vi "Sample Trajectory.vi"(9 "start index (0)":i32, 10 "timestamp":dbl, 11 "Trajectory States":T1[](array[typedef])) -> (1 "index":i32, 2 "State":T1, 3 "Trajectory States out":T1[](array[typedef]))   [LabVIEW 2019]
uses:
  Typedef/Trajectory State.ctl
  Geometry/Typedef/Pose2d.ctl
  Geometry/Typedef/Translation2d.ctl
  Geometry/Typedef/Rotation2d.ctl
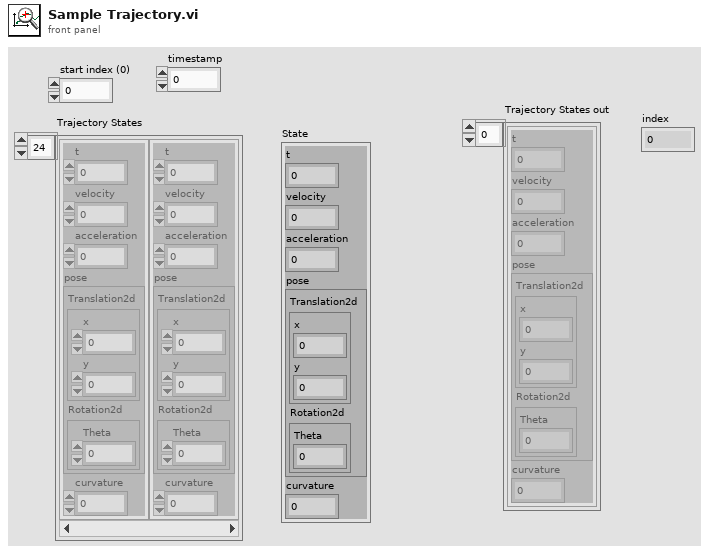
[diagram p1: front panel]
types:
  T1 = typedef "Trajectory State.ctl" = cluster{"t":dbl, "velocity":dbl, "acceleration":dbl, "pose":T2, "curvature":dbl}
  T2 = typedef "Pose2d.ctl" = cluster{"Translation2d":T3, "Rotation2d":T4}
  T3 = typedef "Translation2d.ctl" = cluster{"x":dbl, "y":dbl}
  T4 = typedef "Rotation2d.ctl" = cluster{"Theta":dbl}
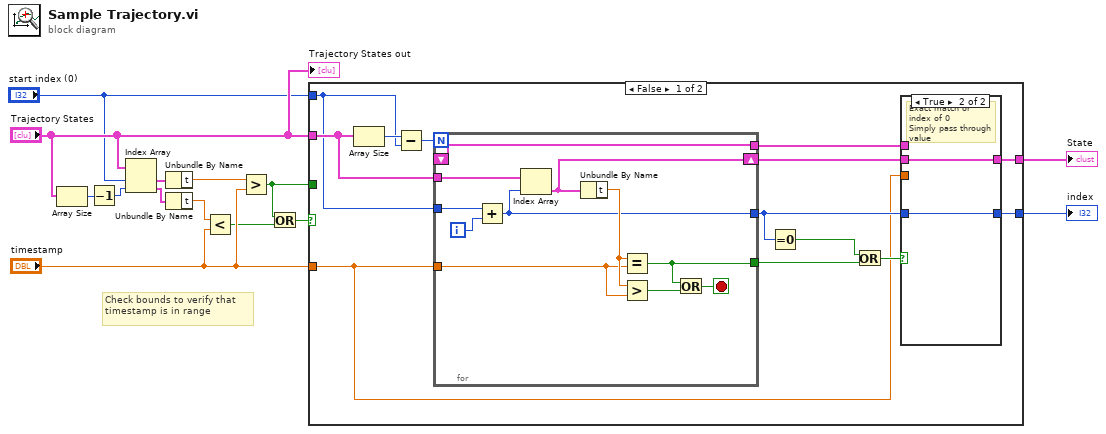
[diagram p0: block diagram]
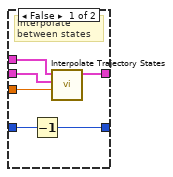
[diagram p2: hidden frame]
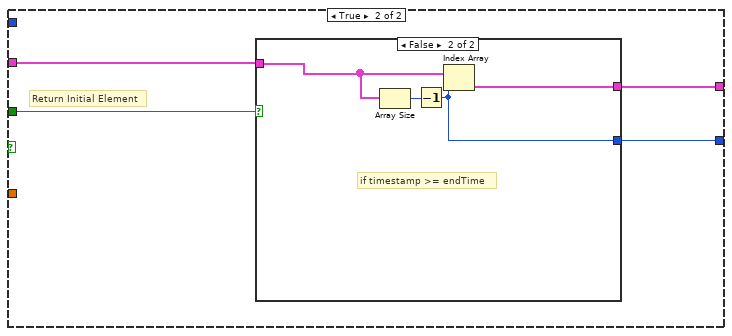
[diagram p3: hidden frame]
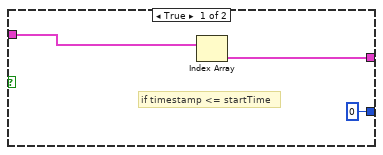
[diagram p4: hidden frame]
diagram:
  # "Check bounds to verify that timestamp is in range"
  n1 = Array Size(array="Trajectory States") -> (size(s)=w12:i32)
  n2 = Decrement(x=w12) -> (x-1=w9:i32)
  n3 = Index Array(array="Trajectory States", index #1="start index (0)", index #2=w9) -> (element #1=w10:T1, element #2=w8:T1)
  n4 = Unbundle By Name(w10) -> ("t"=w5:dbl)
  n5 = Unbundle By Name(w8) -> ("t"=w7:dbl)
  n6 = Less?(x=w7, y="timestamp") -> (x < y?=w1:bool)
  n7 = Greater?(x=w5, y="timestamp") -> (0:w2:bool)
  n8 = Or(x=w2, y=w1) -> (x .or. y?=w3:bool)
  n9 = case shown="False" w3 {
    tunnel: "Trajectory States" -> [w27 w49]
    tunnel: [w20 w48] -> w14
    tunnel: [w18 w47] -> w13
    tunnel: "timestamp" -> [w15 _]
    tunnel: "start index (0)" -> [w16 _]
    tunnel: w2 -> [_ w50]
    frame False {
      n10 = Array Size(array=w27) -> (size(s)=w26:i32)
      n11 = Subtract(x=w26, y=w16) -> (x-y=w25:i32)
      n12 = for {
        N: w25 -> [_]
        tunnel: w27 -> [w38]
        tunnel: w16 -> [w36]
        tunnel: w15 -> [w33]
        tunnel: [w31] -> w24
        shift-right: [w30] -> w21
        shift-left: _ -> [w29]
        tunnel: [w29] -> w17
        tunnel: [w28] -> w19
        i -> [w37]
        stop <- w35 stop-if-true
        n13 = Add(x=w36, y=w37) -> (x+y=w28:i32)
        n14 = Index Array(array=w38, index=w28) -> (element=w30:T1)
        n15 = Unbundle By Name(w30) -> ("t"=w34:dbl)
        n16 = Equal?(x=w34, y=w33) -> (x = y?=w31:bool)
        n17 = Greater?(x=w34, y=w33) -> (0:w32:bool)
        n18 = Or(x=w31, y=w32) -> (x .or. y?=w35:bool)
      }
      n19 = Equal To 0?(x=w19) -> (x = 0?=w23:bool)
      n20 = Or(x=w23, y=w24) -> (x .or. y?=w22:bool)
      n21 = case shown="True" w22 {
        tunnel: w21 -> [w43 w46]
        tunnel: [w42 w46] -> w20
        tunnel: w19 -> [w41 w45]
        tunnel: [w40 w45] -> w18
        tunnel: w17 -> [w44 _]
        tunnel: w15 -> [w39 _]
        frame False {
          # "Interpolate between states"
          n22 = Decrement(x=w41) -> (x-1=w40:i32)
          n23 = call "Interpolate Trajectory States.vi"("timestamp"=w39, "State [n]"=w43, "State [n-1]"=w44) -> ("Interpolated State"=w42:T1)  [unwired: 8 in]
        }
        frame True {
          # "Exact match or index of 0\nSimply pass through value"
        }
      }
    }
    frame True {
      # "Return Initial Element"
      n24 = case shown="False" w50 {
        tunnel: w49 -> [w53 w56]
        tunnel: [w52 w57] -> w48
        tunnel: [0 w54] -> w47
        frame True {
          # "if timestamp <= startTime"
          n25 = Index Array(array=w53) -> (element=w52:T1)  [unwired: 1 in]
        }
        frame False {
          # "if timestamp >= endTime"
          n26 = Array Size(array=w56) -> (size(s)=w55:i32)
          n27 = Decrement(x=w55) -> (x-1=w54:i32)
          n28 = Index Array(array=w56, index=w54) -> (element=w57:T1)
        }
      }
    }
  }
  "State" <- w14
  "index" <- w13
  "Trajectory States out" <- "Trajectory States"
